vi "Simulation.vi"() -> ()   [LabVIEW 2009]
uses:
  <vilib>/Simulation/Scripting/Companion Diagram/SimConfigNode/SimDog.xnode
  <vilib>/Simulation/Implementation/Shared/SIMSCR Execution Mode.ctl
  <vilib>/Simulation/Scripting/Companion Diagram/SimConfigNode/_simSolvers.ctl
  <vilib>/Simulation/Scripting/Companion Diagram/SimConfigNode/SimParams.ctl
  <vilib>/addons/Control Design/_Model Construction/Model Typedefs.llb/CD General Elements.ctl
  <vilib>/addons/Control Design/_Model Construction/NI_LinSys_Model Typedefs.lvlib
  <vilib>/addons/Control Design/_Model Construction/Model Typedefs.llb/CD State Space Model (MIMO).ctl
  <vilib>/Simulation/ContinuousLinear/SIMX StateSpace/SIMX StateSpace.xnode
  <vilib>/Simulation/DataSources/SIMX Step/SIMX Step.xnode
  <vilib>/Simulation/SignalDisplay/SIMX TimeWaveform/SIMX TimeWaveform.xnode
panel:
  out "state_sys":T1 caption="SS object" {"Transport Delay" format="%.2f"; "D" format="%#.2g"; "C" format="%#.2g"; "B" format="%#.2g"; "A" format="%#.2g"; "properties"."Sampling Time" format="%#.6p"; "properties"."Output Delays" format="%.4f"; "properties"."Input Delays" format="%.4f"}
  out "Waveform Chart":waveform(dbl)(graph)
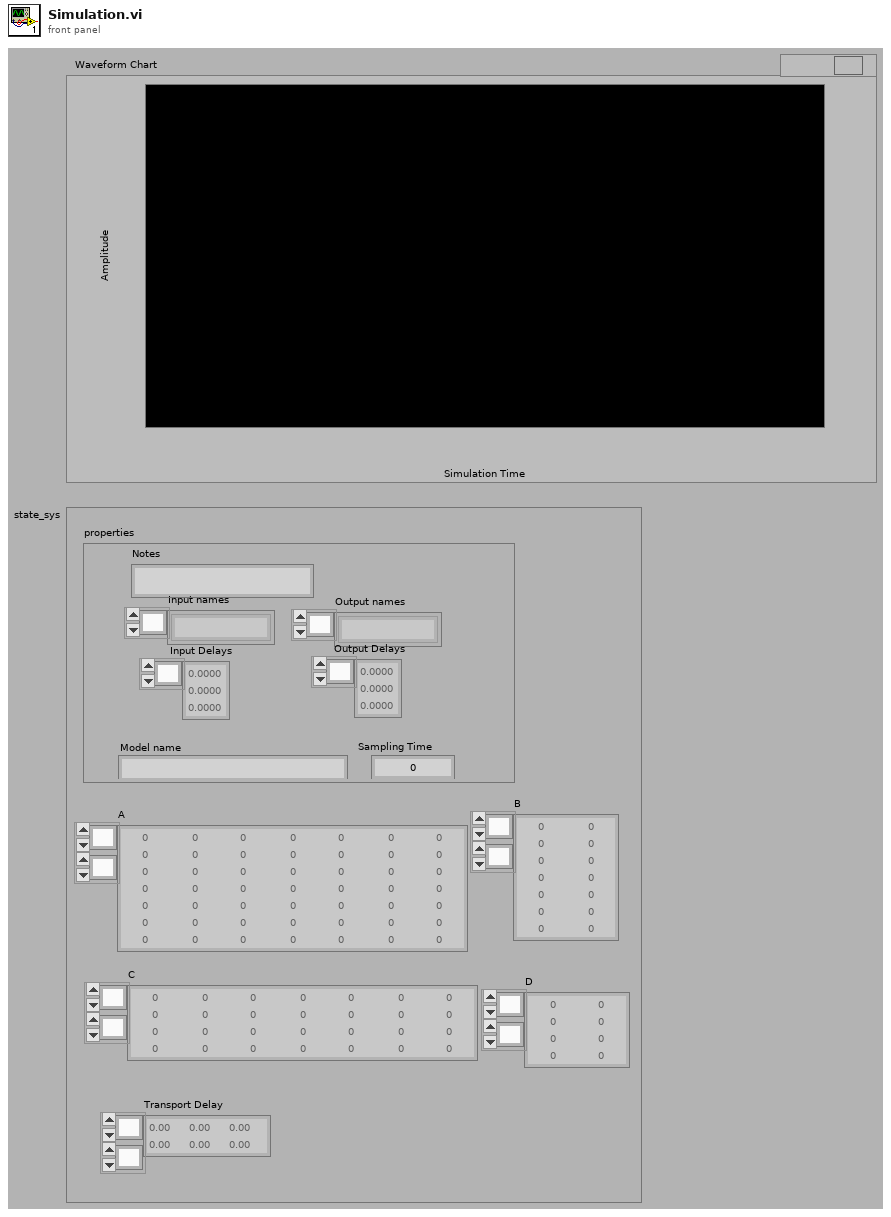
[diagram p1: front panel]
types:
  T1 = typedef "NI_LinSys_Model Typedefs.lvlib/CD State Space Model (MIMO).ctl" = cluster{"properties":T2, "A":dbl[][], "B":dbl[][], "C":dbl[][], "D":dbl[][], "StateNames":string[], "Transport Delay":dbl[][]}
  T2 = typedef "NI_LinSys_Model Typedefs.lvlib/CD General Elements.ctl" = cluster{"Model name":string, "Input names":string[], "Output names":string[], "Input Delays":dbl[], "Output Delays":dbl[], "Sampling Time":dbl, "Notes":string}
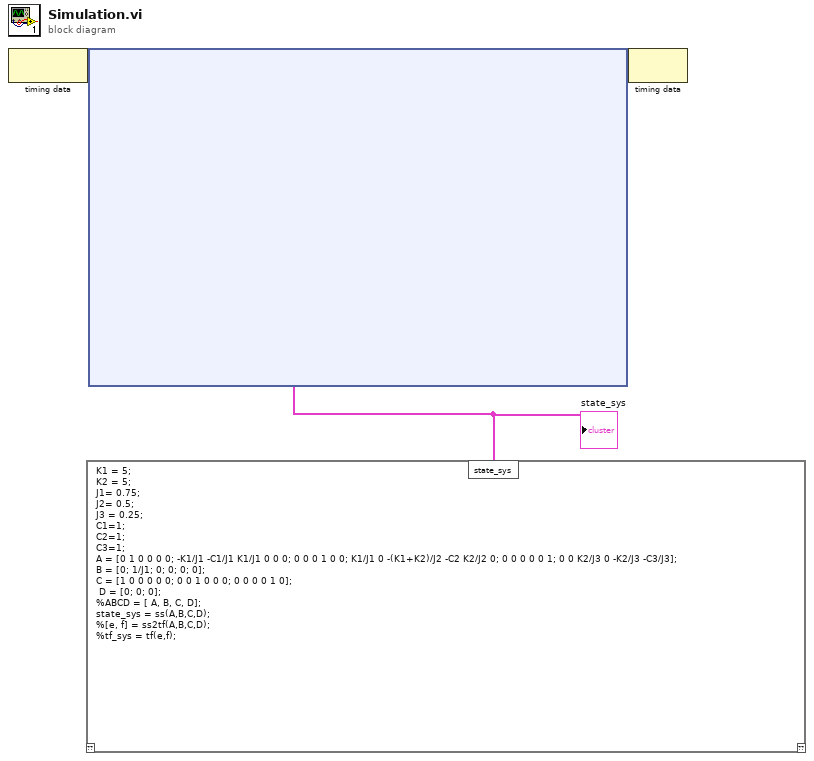
[diagram p0: block diagram]
diagram:
  n1 = node-c288() -> (w3:variant)  [unwired: 1 in]
  n2 = mathscript code="K1 = 5;\nK2 = 5;\nJ1= 0.75;\nJ2= 0.5;\nJ3 = 0.25;\nC1=1;\nC2=1;\nC3=1;\nA = [0 1 0 0 0 0; -K1/J1 -C1/J1 K1/J1 0 0 0; 0 0 0 1 0 0; K1/J1 0 -(K1+K2)/J2 -C2 K2/J2 0; 0 0 0 0 0 1; 0 0 K2/J3 0 -K2/J3 -C3/J3];\nB = [0; 1/J1; 0; 0; 0; 0];\nC = [1 0 0 0 0 0; 0 0 1 0 0 0; 0 0 0 0 1 0];\n D = [0; 0; 0];\n%ABCD = [ A, B, C, D];\nstate_sys = ss(A,B,C,D);\n%[e, f] = ss2tf(A,B,C,D);\n%tf_sys = tf(e,f);"() -> ("state_sys"=w1:T1)  [unwired: 1 in, 1 out]
  "state_sys" <- w1
  n3 = node-c254 ("Control & Simulation Loop")(w3, w1) -> (w2:variant)
  n4 = node-c288(w2) -> ()  [unwired: 1 out]
